vi "OAT Detrend Analog Tacho Signal (N Tachos).vi"(0 "analog tacho signals":waveform(dbl)[](array[waveform]), 1 "extension":T1(ring)=enum."symmetric ext.", 5 "detrend level (0.0)":dbl min=0.0 max=1.0 step=0.01 format="%.2f", 7 "analysis filters":cluster{"lowpass":dbl[], "highpass":dbl[]}={"lowpass"=[0.4829629131445343, 0.8365163037378082, 0.22414386804201325, -0.12940952255126054], "highpass"=[-0.1294095225512602, -0.22414386804201353, 0.8365163037378076, -0.48296291314453393]} {"highpass" format="%.2e"; "lowpass" format="%.2e"}, 9 "synthesis filters":cluster{"lowpass":dbl[], "highpass":dbl[]}={"lowpass"=[-0.1294095225512602, 0.22414386804201353, 0.8365163037378076, 0.48296291314453393], "highpass"=[-0.4829629131445343, 0.8365163037378082, -0.22414386804201325, -0.12940952255126054]} {"highpass" format="%.2e"; "lowpass" format="%.2e"}, 11 "error in (no error)":errorcluster) -> (4 "detrended analog tacho signals":waveform(dbl)[](array[waveform]), 6 "trends":waveform(dbl)[](array[waveform]), 15 "error out":errorcluster)   [LabVIEW 2017, in "SoundVib_TachProcess.lvlib"]
doc: "Removes trend from an analog tachometer signal. You can use the output of this VI as an input for the OAT Analog Tacho Process VI. Wire data to the <B>analog tacho signal</B> input to determine the polymorphic instance to use or manually select the instance."
uses:
  <vilib>/addons/Sound and Vibration/Order Analysis/Tach Process/SoundVib_TachProcess.lvlib
  <resource>/sndvib.dll
panel:
  in  "Array":waveform(dbl)[](array[waveform])
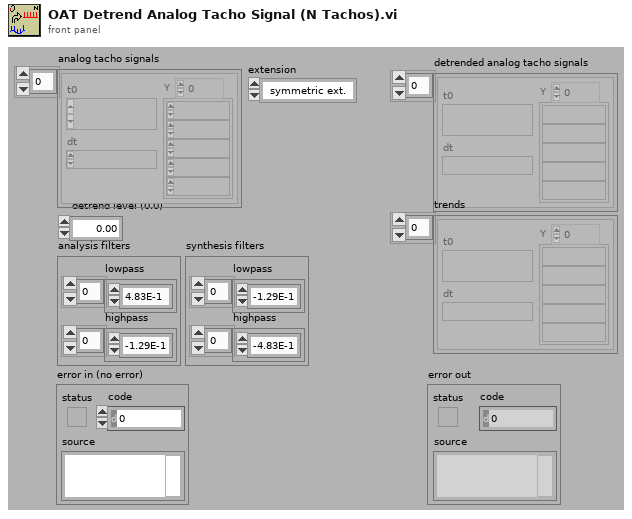
[diagram p1: front panel]
types:
  T1 = enum16{"zero padding", "symmetric ext.", "periodic ext.", "1st derivative", "2nd derivative"}
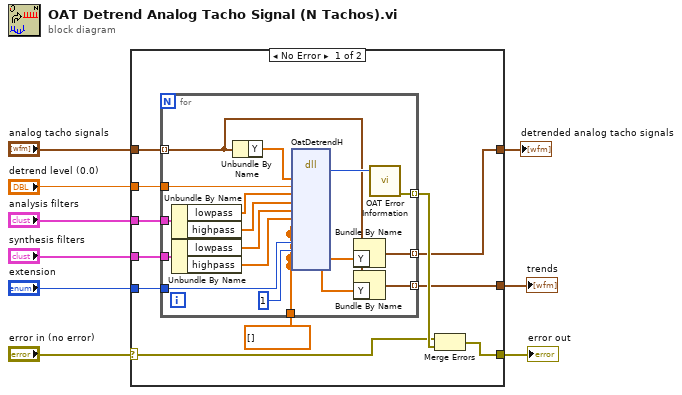
[diagram p0: block diagram]
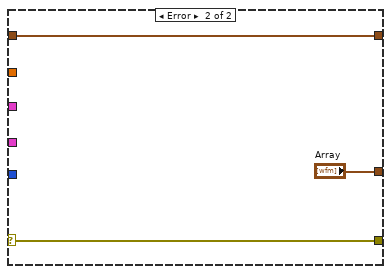
[diagram p2: hidden frame]
diagram:
  n1 = case shown="No Error" "error in (no error)" {
    selector: "error in (no error)" -> [w10 w41]
    tunnel: "detrend level (0.0)" -> [w20 _]
    tunnel: "analysis filters" -> [w19 _]
    tunnel: "synthesis filters" -> [w18 _]
    tunnel: "extension" -> [w17 _]
    tunnel: [w14 w40] -> w5
    tunnel: [w13 "Array"] -> w4
    tunnel: "analog tacho signals" -> [w12 w40]
    tunnel: [w11 w41] -> w2
    frame No Error {
      n2 = for {
        tunnel: w20 -> [w38]
        tunnel: w19 -> [w37]
        tunnel: w18 -> [w34]
        tunnel: w17 -> [w31]
        tunnel: dbl[] [] ("Array") -> [w29]
        tunnel: [w27] -> w15 mode=indexing
        tunnel: [w24] -> w14 mode=indexing
        tunnel: [w23] -> w13 mode=indexing
        tunnel: w12 -> [w21] mode=indexing
        n3 = Unbundle By Name(w37) -> ("lowpass"=w36:dbl[], "highpass"=w35:dbl[])
        n4 = Unbundle By Name(w34) -> ("lowpass"=w33:dbl[], "highpass"=w32:dbl[])
        n5 = Unbundle By Name(w21) -> ("Y"=w26:dbl[])
        n6 = dll-call lib="C:/Program Files (x86)/National Instruments/LabVIEW 2017/resource/sndvib.*" fn="OatDetrendH"("xH"=w26, "level"=w38, "a_lowpassH"=w36, "a_highpassH"=w35, "s_lowpassH"=w33, "s_highpassH"=w32, "initialCondition"=w29, "finalCondition"=w29, "extension"=w31, "shift"=1, "detrendH"=w29, "trendH"=w29) -> ("return type"=w28:i32, "detrendH"=w25:dbl[], "trendH"=w22:dbl[])  [unwired: 13 in, 2 out]
        n7 = Bundle By Name(cluster=w21, "Y"=w25) -> (w24:waveform(dbl))
        n8 = Bundle By Name(cluster=w21, "Y"=w22) -> (w23:waveform(dbl))
        n9 = call <vilib>:"OAT Error Information.vi"("error code"=w28) -> ("error out"=w27:errorcluster)  [unwired: 6 in]
      }
      n10 = Merge Errors(w10, w15) -> (w11:errorcluster)
    }
    frame Error {
    }
  }
  "detrended analog tacho signals" <- w5
  "trends" <- w4
  "error out" <- w2
